vi "实验3.vi"() -> ()   [LabVIEW 2022 SP3]
uses:
  <vilib>/measure/madcrms.llb/Basic Averaged DC-RMS for 1 Chan.vi
  <vilib>/measure/NI_MAPro.lvlib
  <vilib>/gmath/NI_Gmath.lvlib
panel:
  in  "开关":bool
  out "峰峰值（V）":dbl
  out "有效值（V）":dbl
  out "平均值（V）":dbl
  out "直流分量（V）":dbl
  in  "直流 / 交流":bool
  in  "实际 / 仿真":bool
  in  "停止":bool
  in  "波形选择":enum16{"正弦波", "三角波", "方波", "锯齿波"}(ring)
  in  "占空比（%）":i8
  in  "初始相位":sgl
  in  "直流偏移":sgl
  in  "采样频率（Hz）":sgl
  in  "频率（Hz）":dbl
  in  "幅度（V）":sgl
  in  "采样点数":i32
  out "监视器":sgl[](graph)
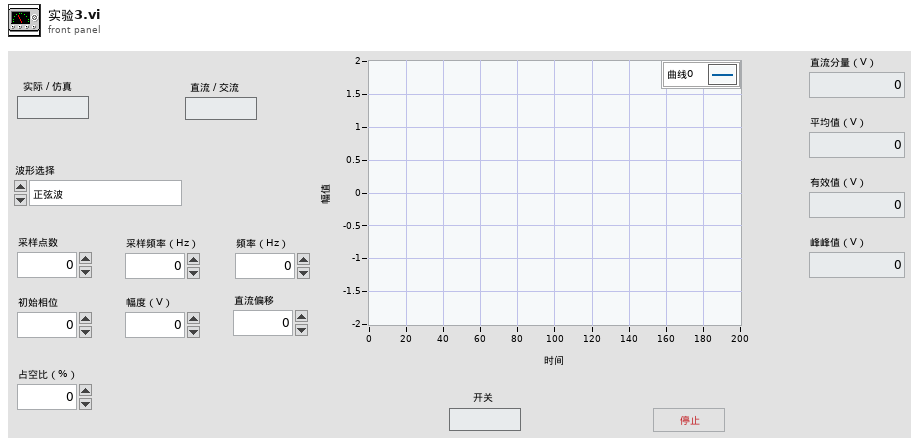
[diagram p1: front panel]
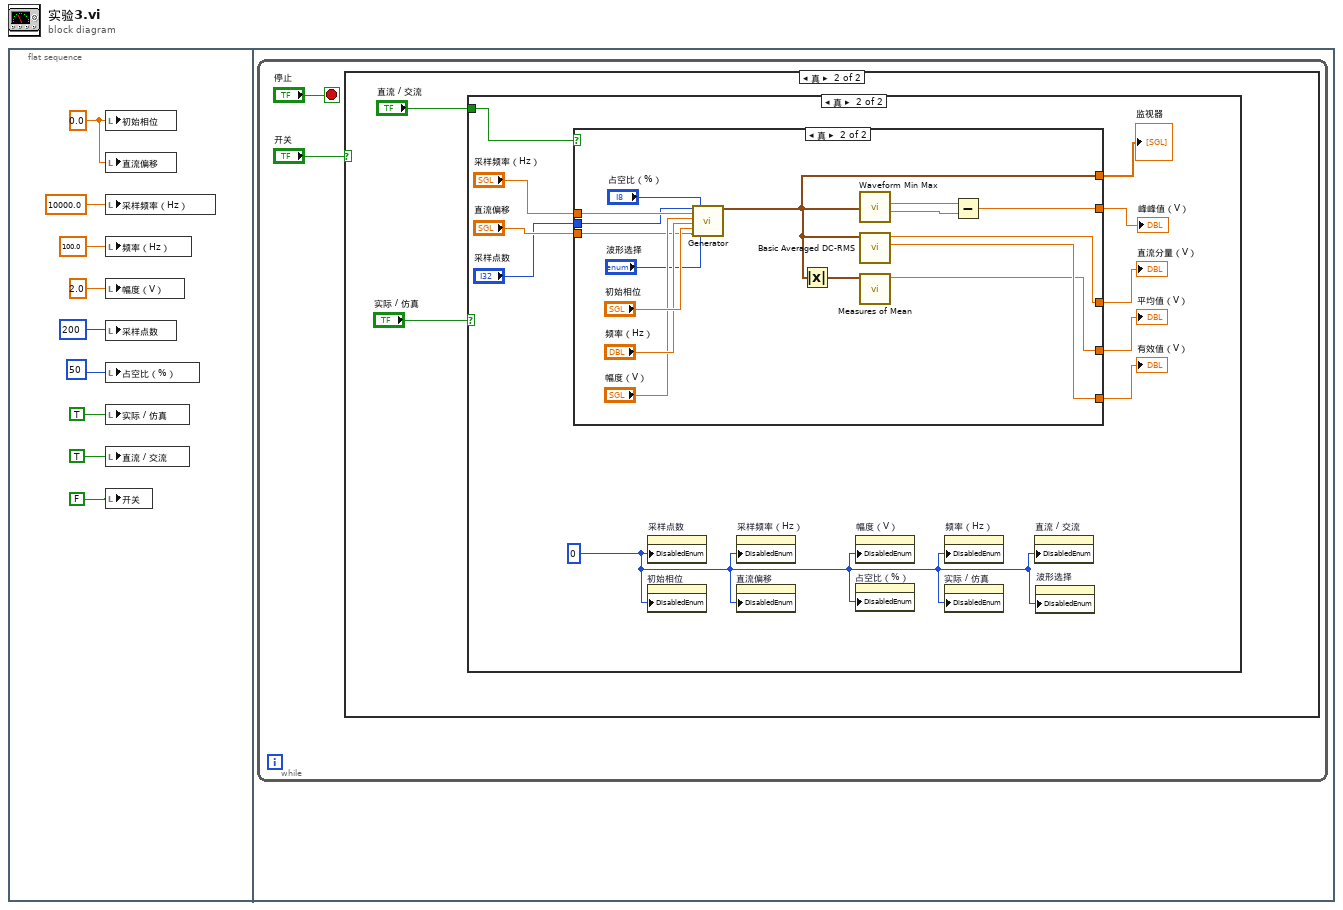
[diagram p0: block diagram]
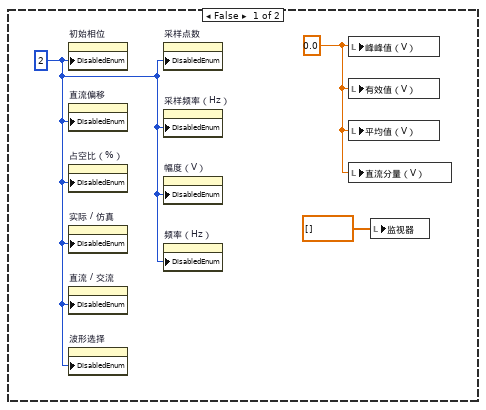
[diagram p2: hidden frame]
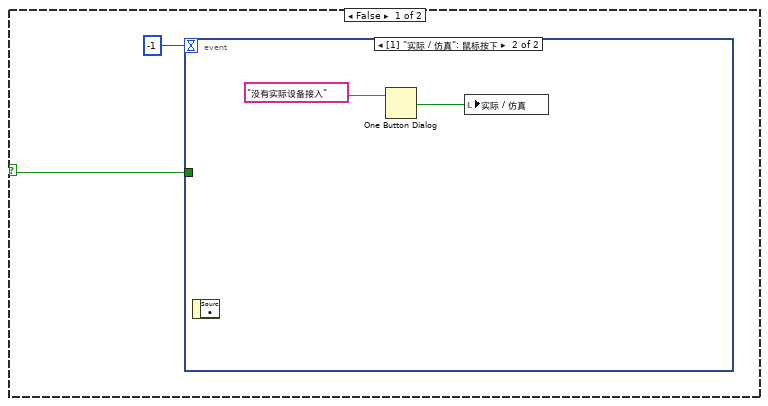
[diagram p3: hidden frame]
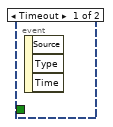
[diagram p4: hidden frame]
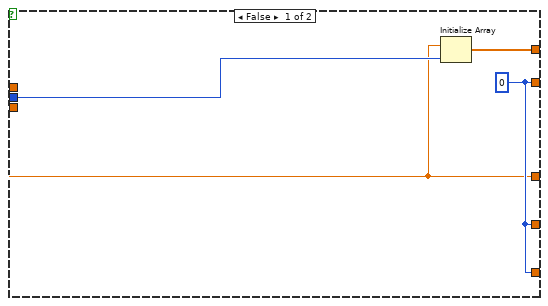
[diagram p5: hidden frame]
diagram:
  n1 = flat-sequence {
    frame #0 {
      w7 = 0.0
      n2 = local write "初始相位"(w7) -> ()
      n3 = local write "直流偏移"(w7) -> ()
      n4 = local write "采样频率（Hz）"(10000.0) -> ()
      n5 = local write "频率（Hz）"(100.0) -> ()
      n6 = local write "幅度（V）"(2.0) -> ()
      n7 = local write "采样点数"(200) -> ()
      n8 = local write "占空比（%）"(50) -> ()
      n9 = local write "实际 / 仿真"(TRUE) -> ()
      n10 = local write "直流 / 交流"(TRUE) -> ()
      n11 = local write "开关"(FALSE) -> ()
    }
    frame #1 {
      n12 = while {
        stop <- "停止" stop-if-true
        n13 = case shown="真" "开关" {
          frame False {
            w12 = 2
            w14 = 0.0
            n14 = property on="初始相位" class="DigNum (严格)"("DisabledEnum"=w12) -> ()  [unwired: 2 in, 2 out]
            n15 = property on="直流偏移" class="DigNum (严格)"("DisabledEnum"=w12) -> ()  [unwired: 2 in, 2 out]
            n16 = property on="占空比（%）" class="DigNum (严格)"("DisabledEnum"=w12) -> ()  [unwired: 2 in, 2 out]
            n17 = property on="实际 / 仿真" class="Bool (严格)"("DisabledEnum"=w12) -> ()  [unwired: 2 in, 2 out]
            n18 = property on="直流 / 交流" class="Bool (严格)"("DisabledEnum"=w12) -> ()  [unwired: 2 in, 2 out]
            n19 = property on="波形选择" class="Enum (严格)"("DisabledEnum"=w12) -> ()  [unwired: 2 in, 2 out]
            n20 = property on="采样点数" class="DigNum (严格)"("DisabledEnum"=w12) -> ()  [unwired: 2 in, 2 out]
            n21 = property on="采样频率（Hz）" class="DigNum (严格)"("DisabledEnum"=w12) -> ()  [unwired: 2 in, 2 out]
            n22 = property on="幅度（V）" class="DigNum (严格)"("DisabledEnum"=w12) -> ()  [unwired: 2 in, 2 out]
            n23 = property on="频率（Hz）" class="DigNum (严格)"("DisabledEnum"=w12) -> ()  [unwired: 2 in, 2 out]
            n24 = local write "峰峰值（V）"(w14) -> ()
            n25 = local write "有效值（V）"(w14) -> ()
            n26 = local write "平均值（V）"(w14) -> ()
            n27 = local write "直流分量（V）"(w14) -> ()
            n28 = local write "监视器"(dbl[] []) -> ()
          }
          frame True {
            n29 = case shown="真" "实际 / 仿真" {
              selector: "实际 / 仿真" -> [w17 _]
              tunnel: "直流 / 交流" -> [_ w30]
              frame False {
                n30 = event shown="[1] \"实际 / 仿真\": 鼠标按下" {
                  selector: _ -> [_ _]
                  dyn-events: _ -> [_ _]
                  timeout: -1 -> [_ _]
                  tunnel: w17 -> [_ _]
                  event Timeout {
                    n31 = event-data() -> ()  [unwired: 1 in, 3 out]
                  }
                  event "实际 / 仿真": Mouse Down {
                    n32 = event-data() -> ()  [unwired: 1 in, 1 out]
                    n33 = One Button Dialog(message="没有实际设备接入") -> (true=w19:bool)  [unwired: 1 in]
                    n34 = local write "实际 / 仿真"(w19) -> ()
                  }
                }
              }
              frame True {
                w21 = 0
                n35 = case shown="真" w30 {
                  tunnel: "采样频率（Hz）" -> [_ w45]
                  tunnel: "直流偏移" -> [w31 w44]
                  tunnel: "采样点数" -> [w32 w43]
                  tunnel: [w33 w39] -> w29
                  tunnel: [w34 w38] -> w28
                  tunnel: [w31 w37] -> w27
                  tunnel: [w34 w36] -> w26
                  tunnel: [w34 w35] -> w25
                  frame False {
                    w34 = 0
                    n36 = Initialize Array(w31, w32) -> (w33:sgl[])
                  }
                  frame True {
                    n37 = call "Generator.vi"("采样点数"=w43, "采样频率（Hz）"=w45, "幅度（V）"="幅度（V）", "频率（Hz）"="频率（Hz）", "初始相位"="初始相位", "直流偏移"=w44, "占空比（%）"="占空比（%）", "波形选择"="波形选择") -> ("监视器"=w39:waveform(dbl))  [unwired: 11 in]
                    n38 = Absolute Value(x=w39) -> (abs(x)=w42:waveform(dbl))
                    n39 = call <vilib>:"Waveform Min Max.vi"("waveform in"=w39) -> ("Y min"=w40:dbl, "Y max"=w41:dbl)  [unwired: 5 in, 4 out]
                    n40 = call-poly <vilib>:"Basic Averaged DC-RMS.vi"("signal in"=w39) -> ("RMS value"=w36:dbl, "DC value"=w37:dbl)  [unwired: 7 in, 2 out]
                    n41 = call <vilib>:"Measures of Mean.vi"("x array"=w42) -> ("mean value"=w35:dbl)  [unwired: 9 in, 1 out]
                    n42 = Subtract(x=w41, y=w40) -> (x-y=w38:dbl)
                  }
                }
                "监视器" <- w29
                "直流分量（V）" <- w27
                "平均值（V）" <- w25
                "有效值（V）" <- w26
                "峰峰值（V）" <- w28
                n43 = property on="采样点数" class="DigNum (严格)"("DisabledEnum"=w21) -> ()  [unwired: 2 in, 2 out]
                n44 = property on="初始相位" class="DigNum (严格)"("DisabledEnum"=w21) -> ()  [unwired: 2 in, 2 out]
                n45 = property on="采样频率（Hz）" class="DigNum (严格)"("DisabledEnum"=w21) -> ()  [unwired: 2 in, 2 out]
                n46 = property on="直流偏移" class="DigNum (严格)"("DisabledEnum"=w21) -> ()  [unwired: 2 in, 2 out]
                n47 = property on="幅度（V）" class="DigNum (严格)"("DisabledEnum"=w21) -> ()  [unwired: 2 in, 2 out]
                n48 = property on="占空比（%）" class="DigNum (严格)"("DisabledEnum"=w21) -> ()  [unwired: 2 in, 2 out]
                n49 = property on="频率（Hz）" class="DigNum (严格)"("DisabledEnum"=w21) -> ()  [unwired: 2 in, 2 out]
                n50 = property on="实际 / 仿真" class="Bool (严格)"("DisabledEnum"=w21) -> ()  [unwired: 2 in, 2 out]
                n51 = property on="直流 / 交流" class="Bool (严格)"("DisabledEnum"=w21) -> ()  [unwired: 2 in, 2 out]
                n52 = property on="波形选择" class="Enum (严格)"("DisabledEnum"=w21) -> ()  [unwired: 2 in, 2 out]
              }
            }
          }
        }
      }
    }
  }
